vi "Stop Calculation.vi"(8 "error in (no error)":errorcluster, 11 "CPU FFT Calculator in":refnum<class "CPU FFT Calculator.lvclass">) -> (0 "error out":errorcluster, 3 "CPU FFT Calculator out":refnum<class "CPU FFT Calculator.lvclass">)   [LabVIEW 2020, in "CPU FFT Calculator.lvlib" / "CPU FFT Calculator.lvclass"]
uses:
  CPU FFT Calculator.lvclass
  C:/Users/natan/Documents/G2CPU-Performance-Demo/Calculation Worker/Calculation Worker/Calculation Worker.lvclass
  C:/Program Files/National Instruments/LabVIEW 2026/vi.lib/ActorFramework/Actor/Actor.lvclass
  <vilib>/ActorFramework/Actor/Actor.lvclass/Actor.ctl
  <vilib>/ActorFramework/Message Enqueuer/Message Enqueuer.lvclass/Message Enqueuer.ctl
  Application Manager/Application Manager Messages/Set UI CPU Done Msg/Set UI CPU Done Msg.lvclass/Set UI CPU Done Msg.ctl
  <vilib>/ActorFramework/Message Enqueuer/Init from Existing Queue.vi
  <vilib>/ActorFramework/Message Enqueuer/Enqueue.vi
  Application Manager/Application Manager Messages/Set UI CPU Done Msg/Set UI CPU Done Msg.lvclass
  C:/Program Files/National Instruments/LabVIEW 2026/vi.lib/ActorFramework/Message/Message.lvclass
  CPU FFT Calculator Messages/Start Calculation Msg/Start Calculation Msg.lvclass
  <vilib>/ActorFramework/Message Priority Queue/Priority Enqueue.vi
  <vilib>/ActorFramework/Message Enqueuer/Message Enqueuer.lvclass
  <vilib>/ActorFramework/Actor/Actor.lvclass
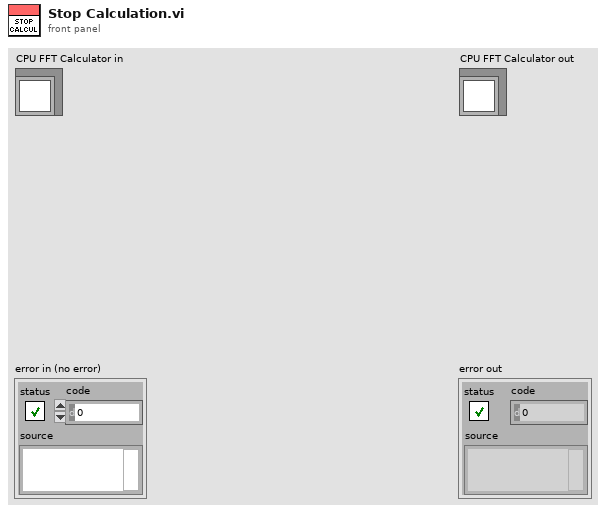
[diagram p1: front panel]
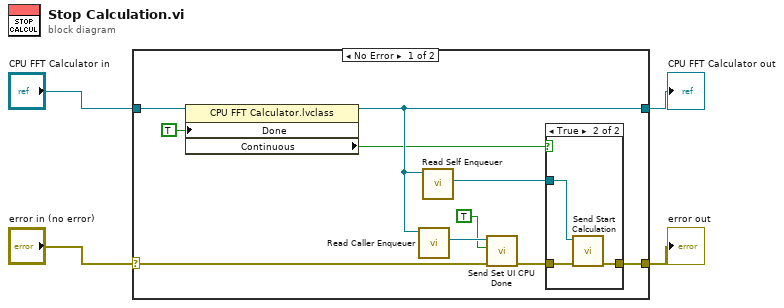
[diagram p0: block diagram]
diagram:
  n1 = case shown="No Error" "error in (no error)" {
    selector: "error in (no error)" -> [w10 w20]
    tunnel: [w6 w20] -> w3
    tunnel: [w9 w19] -> w1
    tunnel: "CPU FFT Calculator in" -> [w14 w19]
    frame No Error {
      n2 = property class="CPU FFT Calculator.lvclass"(reference=w14, "Done"=TRUE) -> (reference out=w9:refnum<class "CPU FFT Calculator.lvclass">, "Continuous"=w5:bool)  [unwired: 1 in, 1 out]
      n3 = call <vilib>:"Read Caller Enqueuer.vi"("Actor"=w9) -> ("Caller Enqueuer"=w12:refnum<class "Message Enqueuer.lvclass">)  [unwired: 10 in]
      n4 = call <vilib>:"Read Self Enqueuer.vi"("Actor"=w9) -> ("Self Enqueuer"=w7:refnum<class "Message Enqueuer.lvclass">)  [unwired: 10 in]
      n5 = call "Send Set UI CPU Done.vi"("error in (no error)"=w10, "CPU Done"=TRUE, "Message Enqueuer"=w12) -> ("error out"=w8:errorcluster)  [unwired: 7 in, 1 out]
      n6 = case shown="True" w5 {
        tunnel: w8 -> [w15 w18]
        tunnel: w7 -> [_ w17]
        tunnel: [w15 w16] -> w6
        frame False {
        }
        frame True {
          n7 = call "Send Start Calculation.vi"("error in (no error)"=w18, "Message Enqueuer"=w17) -> ("error out"=w16:errorcluster)  [unwired: 8 in, 1 out]
        }
      }
    }
    frame Error {
    }
  }
  "error out" <- w3
  "CPU FFT Calculator out" <- w1
